vi "test Empty Array.vi"(8 "error in (no error)":errorcluster, 11 "TestCase in":refnum<class "Data Structure Tests.lvclass">) -> (0 "error out":errorcluster, 3 "TestCase out":refnum<class "Data Structure Tests.lvclass">)   [LabVIEW 2020, in "Data Structure Tests.lvclass"]
uses:
  Data Structure Tests.lvclass
  Data Structure Tests.lvclass/Data Structure Tests.ctl
  <vilib>/addons/_JKI Toolkits/VI Tester/TestCase.llb/TestCase.lvclass
  C:/Program Files/National Instruments/LabVIEW 2020/vi.lib/addons/_JKI Toolkits/VI Tester/TestCase.llb/TestCase.lvclass
  C:/Users/JamesMcNally/Documents/RustInterop/Rust-LabVIEW-Interop/labview-test-project/Data Structure Tests/Data Structure Tests.lvclass
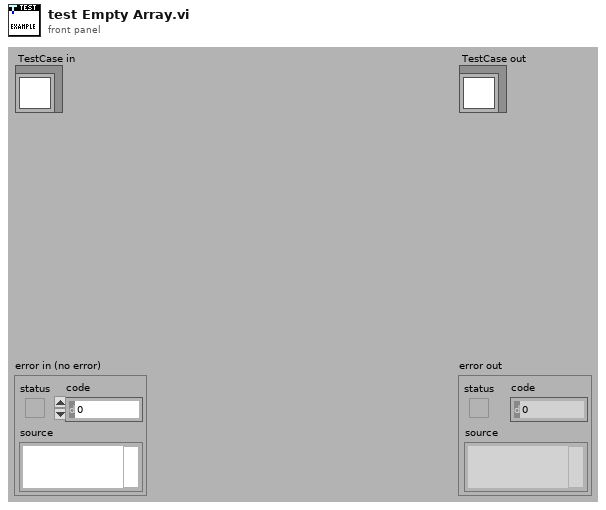
[diagram p1: front panel]
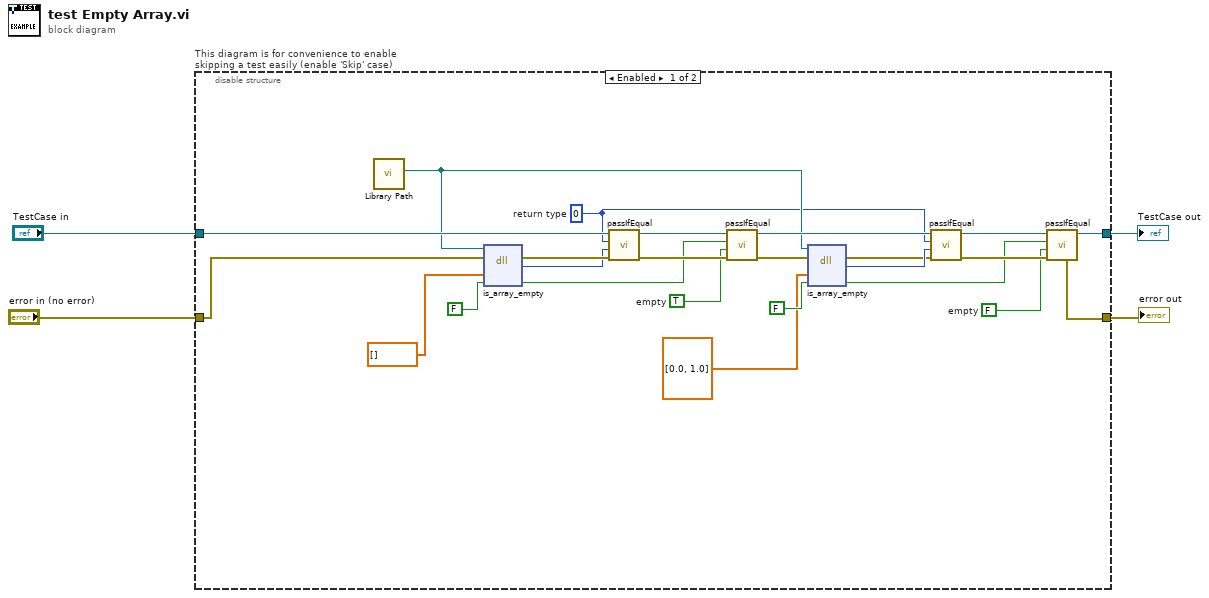
[diagram p0: block diagram]
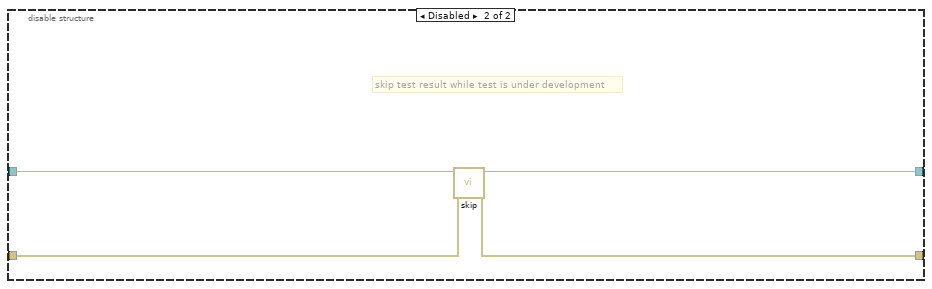
[diagram p2: hidden frame]
diagram:
  n1 = disable-structure "This diagram is for convenience to enable skipping a test easily (enable 'Skip' case)" shown="Enabled" {
    disable-tunnel: "TestCase in" -> [w20 w32]
    disable-tunnel: [w23 w30] -> w1
    disable-tunnel: [w25 w31] -> w3
    disable-tunnel: "error in (no error)" -> [w28 w29]
    frame Enabled {
      w7 = FALSE  # empty
      w8 = TRUE  # empty
      w5 = 0  # return type
      n2 = call "Library Path.vi"() -> ("Library Path"=w10:path)  [unwired: 11 in]
      n3 = dll-call lib="C:/Users/JamesMcNally/Documents/RustInterop/Rust-LabVIEW-Interop/target/debug/labview_test_library.dll" fn="is_array_empty"(path in=w10, error in=w28, "array"=dbl[] [], "empty"=FALSE) -> (error out=w27:errorcluster, "return type"=w16:i32, "empty"=w17:bool)  [unwired: 2 in, 1 out]
      n4 = call-dynamic "passIfEqual.vi"("error in (no error)"=w27, "y"=w16, "x"=w5, "TestCase in"=w20) -> ("error out"=w21:errorcluster, "TestCase out"=w19:refnum<class "Data Structure Tests.lvclass">)  [unwired: 6 in]
      n5 = call-dynamic "passIfEqual.vi"("error in (no error)"=w21, "y"=w8, "x"=w17, "TestCase in"=w19) -> ("error out"=w15:errorcluster, "TestCase out"=w22:refnum<class "Data Structure Tests.lvclass">)  [unwired: 6 in]
      n6 = dll-call lib="C:/Users/JamesMcNally/Documents/RustInterop/Rust-LabVIEW-Interop/target/debug/labview_test_library.dll" fn="is_array_empty"(path in=w10, error in=w15, "array"=dbl[] [0.0, 1.0], "x"=FALSE) -> (error out=w11:errorcluster, "return type"=w14:i32, "x"=w13:bool)  [unwired: 2 in, 1 out]
      n7 = call-dynamic "passIfEqual.vi"("error in (no error)"=w11, "y"=w14, "x"=w5, "TestCase in"=w22) -> ("error out"=w26:errorcluster, "TestCase out"=w24:refnum<class "Data Structure Tests.lvclass">)  [unwired: 6 in]
      n8 = call-dynamic "passIfEqual.vi"("error in (no error)"=w26, "y"=w7, "x"=w13, "TestCase in"=w24) -> ("error out"=w25:errorcluster, "TestCase out"=w23:refnum<class "Data Structure Tests.lvclass">)  [unwired: 6 in]
    }
    frame Disabled {
      # "skip test result while test is under development"
      n9 = call <vilib>:"skip.vi"("error in (no error)"=w29, "TestCase in"=w32) -> ("error out"=w31:errorcluster, "TestCase out"=w30:refnum<class "Data Structure Tests.lvclass">)  [unwired: 8 in]
    }
  }
  "error out" <- w3
  "TestCase out" <- w1
